vi "commander8.vi"() -> ()   [LabVIEW 2015]
uses:
  G_DATA.vi
  G_LCM.vi
  G_VEH.vi
  G_NAV.vi
  G_PATH.vi
  <vilib>/addons/control/pid/pid.llb/PID (DBL).vi
  G_SEN.vi
  <vilib>/addons/control/pid/NI_PID_pid.lvlib
panel:
  in  "handle":dbl
  in  "shifthold":dbl=0.02
  out "String":string="콜 서비스 대기 중"
  out "EURECAR_VISION":T1
  out "count":i32
  out "P2V Sign":picture[](array[picture])=[bytes[7530], bytes[7530], bytes[7530], bytes[7530]]
  out "Array 2":picture[](array[picture])
  out "sign 2":picture[](array[picture])
  out "sign":picture[](array[picture])
  in  "TTL":bool
  in  "Steering gain":dbl=0.8
  out "obs shift":dbl format="%.2f"
  in  "lane keep":bool
  in  "replay":bool
  in  "x":dbl min=-5.0 max=5.0 step=1.0
  out "display":u32=10
  out "control":u32=10
  out "update":bool=TRUE
  in  "save lcm":bool
  out "LCM Recv Data":string="GGA_2\t266\rSDT_GPS_DATA\t268\rGGA_1\t268\rRMC_2\t259\rRMC_1\t262\rEYE_RAW_T\t537\rPATH_T\t1344\rIBEO_2202_T\t672\rPOS_T\t3572\rCON_T\t4009\rCAN_T\t4707\r"
  out "GPS DATA 2":T2={"type"="WAAS", "x_lcc"=-395.2637182511565, "y_lcc"=-852.8277788987846, "latdev"=0.99, "londev"=0.99, "sats"=11, "gps_l1_ranges"=0, "gps_l1_mask_ranges"=0, "gps_l2_mask_ranges"=0, "Heading"=151.74409645131422, "lon"=127.35651, "lat"=36.36776, "time"="15:03:34.8", "hgps"=151.54, "lag"=0.0, "MAP"="KAIST"} {"lag" format="%#_5g"; "hgps" format="%#_5g"; "lat" format="%#_11g"; "lon" format="%#_11g"; "Heading" format="%#_5g"; "latdev" format="%#_4g"; "londev" format="%#_4g"}
  in  "Obs":bool=TRUE
  in  "Log":bool
  out "path":u32=10
  out "sensor":u32=10 format="%02.0f"
  out "Speed limit":dbl=20.0
  out "collision":bool
  in  "Load Path":bool
  in  "Max. Vel.":dbl=20.0 min=-5.0 max=120.0 step=5.0
  in  "RESET PATH":bool
  out "col":i16(graph)
  out "stop":bool
  in  "Reverse":bool
  in  "STOP":bool
  out "Waveform Chart 4":cluster{"auto":i16, "run":i16}(graph)={"auto"=1, "run"=0}
  out "Waveform Chart 3":cluster{"Steer_input":dbl, dbl, "handle":dbl}(graph)
  out "Waveform Chart 2":T3(graph)={"VS_des"=0.0, "VS_can"=31.498562500000002, "VS_des"=20.0}
  out "Heading":cluster{"Heading":dbl, "hgps":dbl}(graph)={"Heading"=151.74409645131422, "hgps"=151.54}
  out "XY Graph 2":cluster{"Y":dbl[], "Y":dbl[]}[](graph)=[{"Y"=[-395.3040396828474], "Y"=[-852.7527551292769]}, {"Y"=array[29298 elements], "Y"=array[29298 elements]}, {"Y"=array[29298 elements], "Y"=array[29298 elements]}, {"Y"=[-390.58210518912017], "Y"=[-861.284610912867]}]
  out "Gauge":cluster{dbl, dbl, dbl}(knob)={0.0, 31.498562500000002, 20.0} scale=-20.0..140.0
  out "Meter":cluster{dbl, dbl, dbl}(knob)={-3.5333877271700453, -5.2, -7.217874503679048} scale=-550.0..550.0
  out "XY Graph":cluster{"Y":dbl[], "Y":dbl[]}[](graph)=[{"Y"=array[11233 elements], "Y"=array[11233 elements]}, {"Y"=[-0.0, 0.0027755521495791413, 0.011103235155417224, 0.024986130588096955, 0.04442938073793812, 0.0694401981527264, 0.10002787904836907, 0.13620382065079895, 0.17798154254490584, 0.22537671212434418, 0.2784071742547809, 0.3370929852830926, 0.40145645154536425, 0.4715221725490224, 0.5473170890276435, 0.6288705360921867, 0.7162143017295008, 0.8093826909282242, 0.9084125957438758, 1.0133435716494645, 1.1242179205557647, 1.2410807809266515, 1.3639802254602955, 1.4929673668571652, 1.6280964722509026, 1.769425086939485, 1.9170141681219874, 2.0709282294217246, 2.2312354970611636, 2.3980080786478197, 2.5713221456362234], "Y"=[0.0, 0.5, 1.0, 1.5, 2.0, 2.5, 3.0, 3.5, 4.0, 4.5, 5.0, 5.5, 6.0, 6.5, 7.0, 7.5, 8.0, 8.5, 9.0, 9.5, 10.0, 10.5, 11.0, 11.5, 12.0, 12.5, 13.0, 13.5, 14.0, 14.5, 15.0]}, {"Y"=[-0.40885366553013214], "Y"=[0.1442103688222703]}, {"Y"=array[212 elements], "Y"=array[212 elements]}, {"Y"=[-0.925, -0.925, -0.925, -0.6775, -0.6775, -0.925, -0.925, -0.925, -0.925, -0.6775, -0.6775, -0.925, -0.925, -0.925, 0.9025, 0.9025, 0.9025, 0.6775, 0.6775, 0.9025, 0.9025, 0.9025, 0.9025, 0.6775, 0.6775, 0.9025, 0.9025, 0.9025, -0.925], "Y"=[-0.75, -0.224, 0.224, 0.224, -0.224, -0.224, 0.224, 2.415, 2.885, 2.885, 2.415, 2.415, 2.885, 3.5, 3.5, 2.885, 2.415, 2.415, 2.885, 2.885, 2.415, 0.224, -0.224, -0.224, 0.224, 0.224, -0.224, -0.75, -0.75]}, {"Y"=[0.0, 0.0, 0.0, 0.0, 0.0, 0.0, 0.0, 0.0, 0.0, 0.0], "Y"=[0.0, 0.5, 1.0, 1.5, 2.0, 2.5, 3.0, 3.5, 4.0, 4.5]}, {"Y"=[1.41796875, 1.3798326583616436, 1.3415997434556484, 1.3032752327956258, 1.2648643538951874, 1.226372334267944, 1.1878044014275073, 1.1491657828874886, 1.110461706161499, 1.07169739876315], "Y"=[0.0, 0.5, 1.0, 1.5, 2.0, 2.5, 3.0, 3.5, 4.0, 4.5]}, {"Y"=[-2.5234375, -2.5105986626297234, -2.4915998479127883, -2.466420726940036, -2.4350409708023073, -2.3974402505904435, -2.3535982373952864, -2.303494602307677, -2.247109016418457, -2.184421150818467], "Y"=[0.0, 0.5, 1.0, 1.5, 2.0, 2.5, 3.0, 3.5, 4.0, 4.5]}, {"Y"=[0.0, 0.0, 0.0, 0.0, 0.0, 0.0, 0.0, 0.0, 0.0, 0.0, 0.0, 0.0, 0.0, 0.0, 0.0, 0.0, 0.0, 0.0, 0.0, 0.0], "Y"=[0.0, 0.5, 1.0, 1.5, 2.0, 2.5, 3.0, 3.5, 4.0, 4.5, 5.0, 5.5, 6.0, 6.5, 7.0, 7.5, 8.0, 8.5, 9.0, 9.5]}]
  in  "Make WPT":bool
  # "e"
  # "V2I Traffic Signal"
  # "CNN\nSign\nDetection"
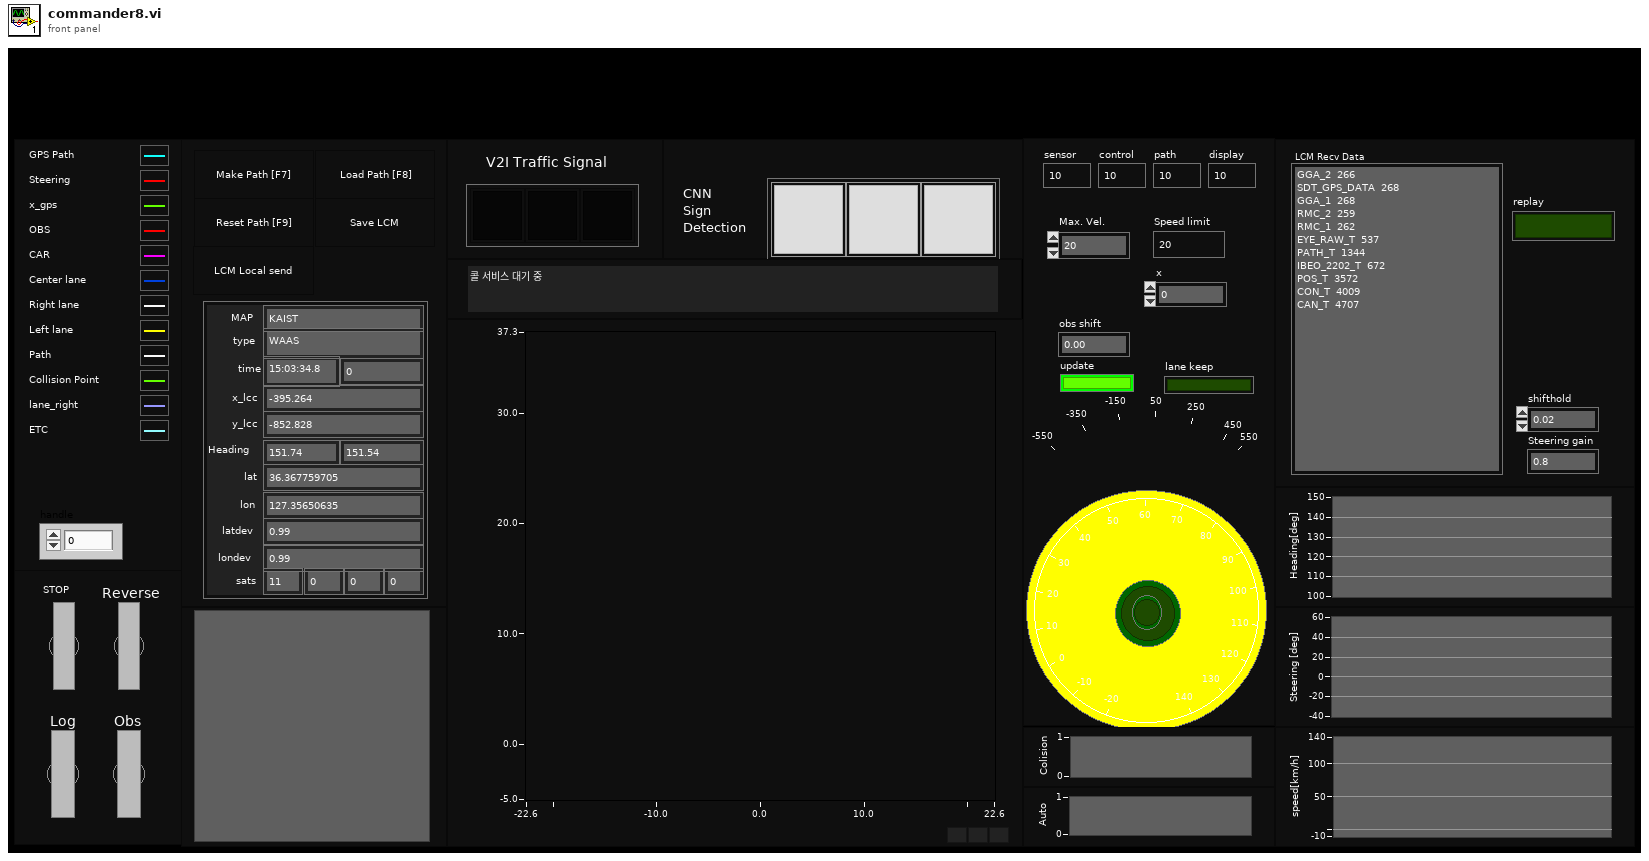
[diagram p1: front panel]
types:
  T1 = cluster{"hash":i64, "sys time":i64, "status":i32, "TS_num":i32, "TS_type":i32[], "TS_loc_x":dbl[], "TS_loc_y":dbl[]}
  T2 = cluster{"type":string, "x_lcc":dbl, "y_lcc":dbl, "latdev":sgl, "londev":sgl, "sats":u8, "gps_l1_ranges":u8, "gps_l1_mask_ranges":u8, "gps_l2_mask_ranges":u8, "Heading":dbl, "lon":sgl, "lat":sgl, "time":string, "hgps":dbl, "lag":dbl, "MAP":string}
  T3 = cluster{"VS_des":dbl, "VS_can":dbl, "VS_des":dbl}
  T4 = enum8{"Enabled", "Disabled", "Disabled and Grayed Out"}
  T5 = cluster{"proportional gain (Kc)":dbl, "integral time (Ti, min)":dbl, "derivative time (Td, min)":dbl}
  T6 = cluster{"idx":i32, "x":dbl, "y":dbl, "h":dbl, "x_path":dbl}
  T7 = cluster{"idx":i32, "x":dbl, "y":dbl, "hp":dbl, "x_path":dbl}
  T8 = cluster{"Steer_input":dbl, "Steer_output":dbl, "VS_des":dbl, "VS_can":dbl, "heading":dbl, "auto":bool, "run":bool, "x":dbl, "y":dbl}
  T9 = cluster{"GPSTime":dbl, "attitude[2]":dbl, "lcc[0]":dbl, "lcc[1]":dbl, "heading_GPS":dbl}
  T10 = cluster{"X":cluster{"idx":i32, "x":dbl, "y":dbl, "h":dbl, "x_path":dbl}}[]
  T11 = typedef "imagedata.ctl" = cluster{"image type":i32, "image depth":i32, "image":u8[], "mask":u8[], "colors":u32[], "Rectangle":cluster{"left":i16, "top":i16, "right":i16, "bottom":i16}}
  T12 = cluster{"hash":i64, "sys time":i64, "s_lat":dbl, "s_lon":dbl, "d_lat":dbl, "d_lon":dbl, "Message":i64}
  T13 = cluster{"Minimum":dbl, "Minimum":dbl, "Minimum":dbl, "Minimum":dbl, "Minimum":dbl}
  T14 = cluster{"X":cluster{"c_idx":i32, "xc":dbl, "yc":dbl, "hc":dbl, "xc_path":dbl}}[]
  T15 = cluster{"hash":i64, "sys time":i64, "time":dbl, "x":dbl, "y":dbl, "h":dbl, "numSV":i32, "postype":i32, "lag":i32, "hordev":dbl, "lat":dbl, "lon":dbl, "hgt":dbl, "map_idx":i32}
  T16 = cluster{"identifier":u32, "timestamp":timestamp, "payload":u8[]}
  T17 = cluster{"hash":i64, "sys time":i64, "size":i32, "data":u8[]}
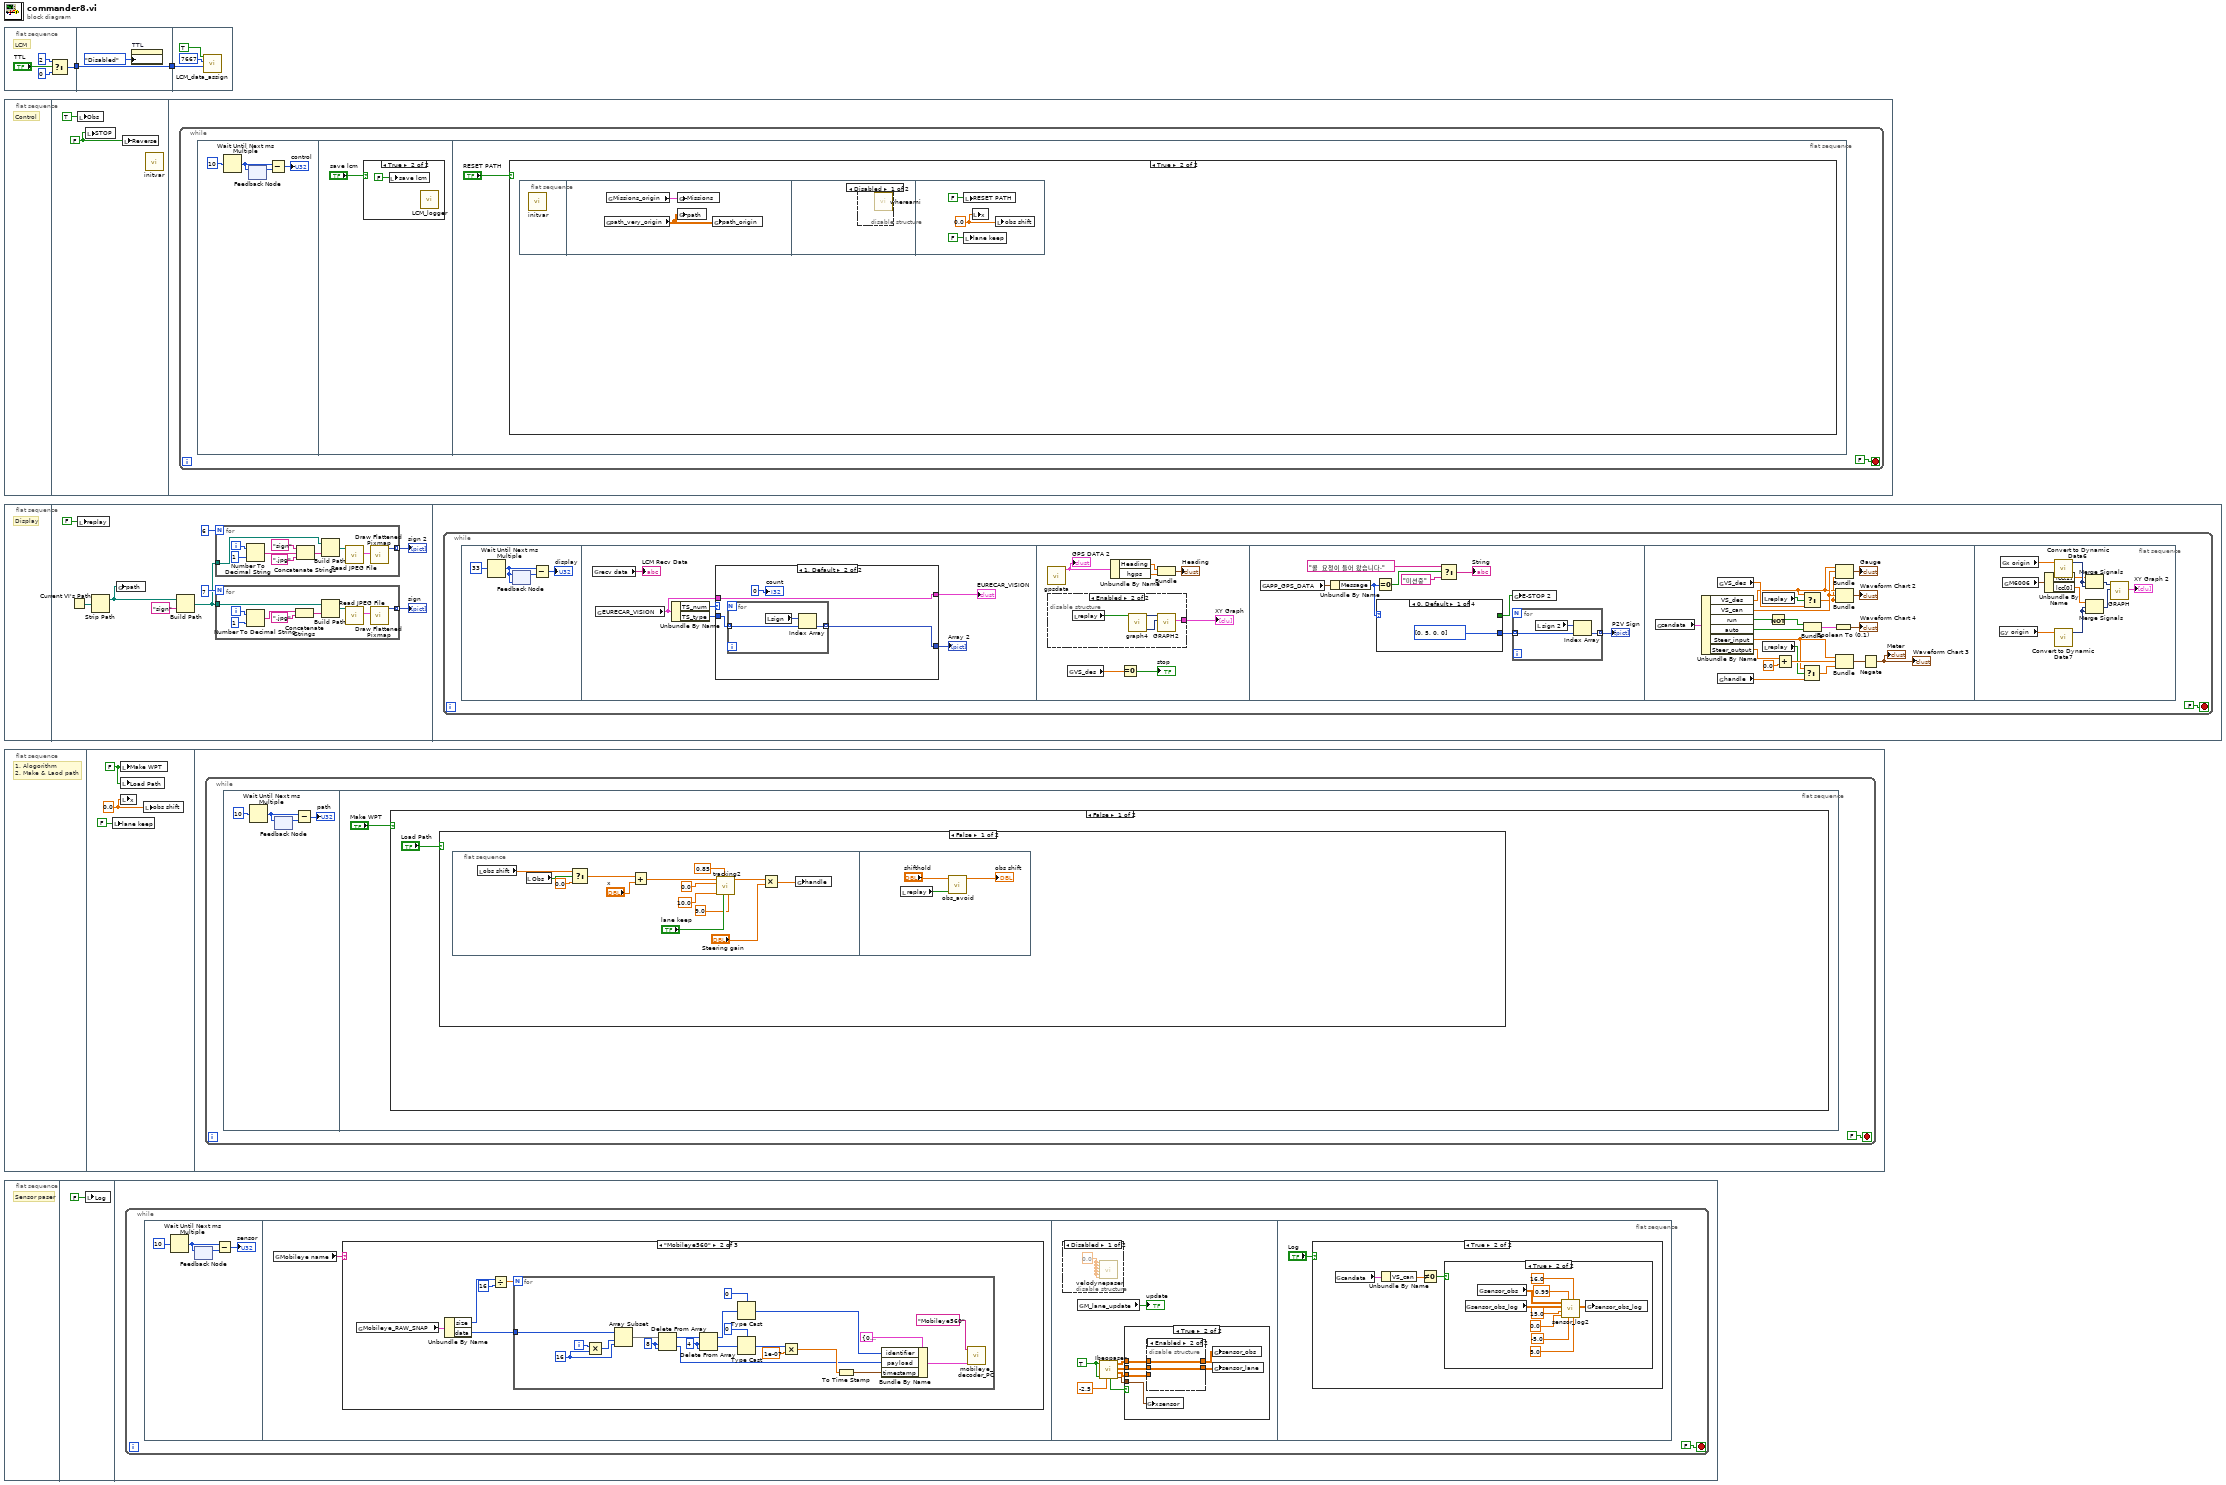
[diagram p0: block diagram]
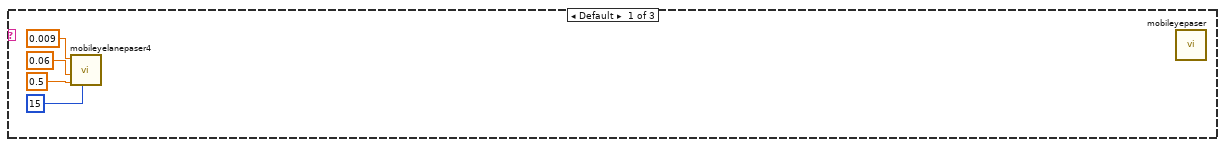
[diagram p2: hidden frame]
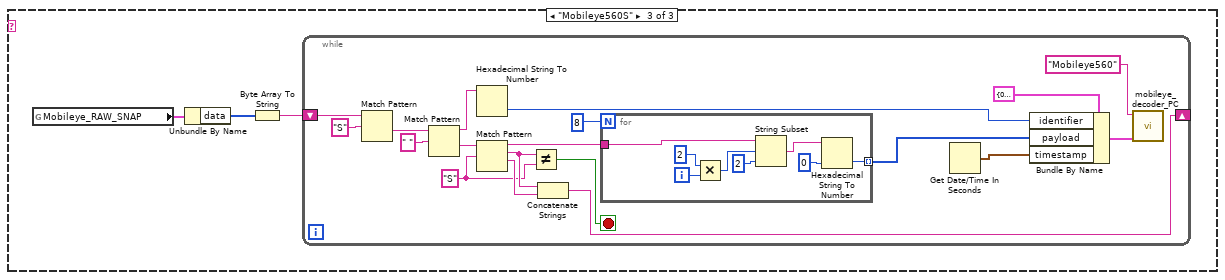
[diagram p3: hidden frame]
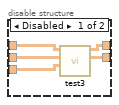
[diagram p6: hidden frame]
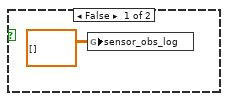
[diagram p7: hidden frame]
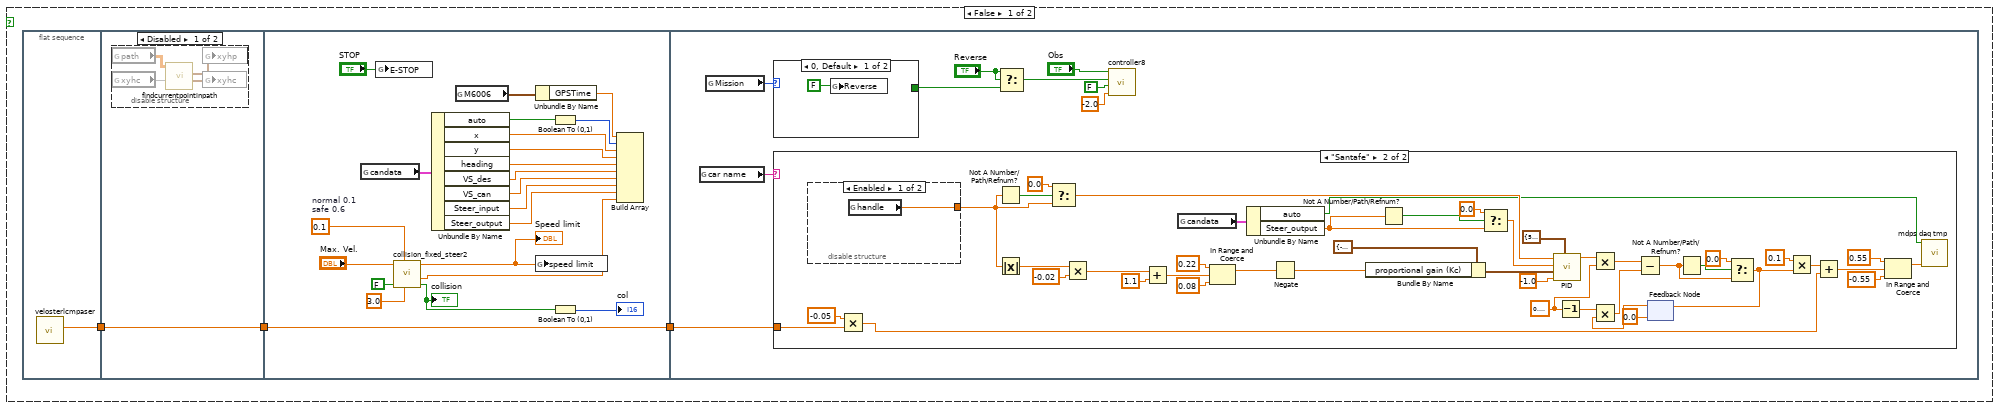
[diagram p10: hidden frame]
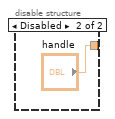
[diagram p13: hidden frame]
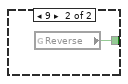
[diagram p14: hidden frame]
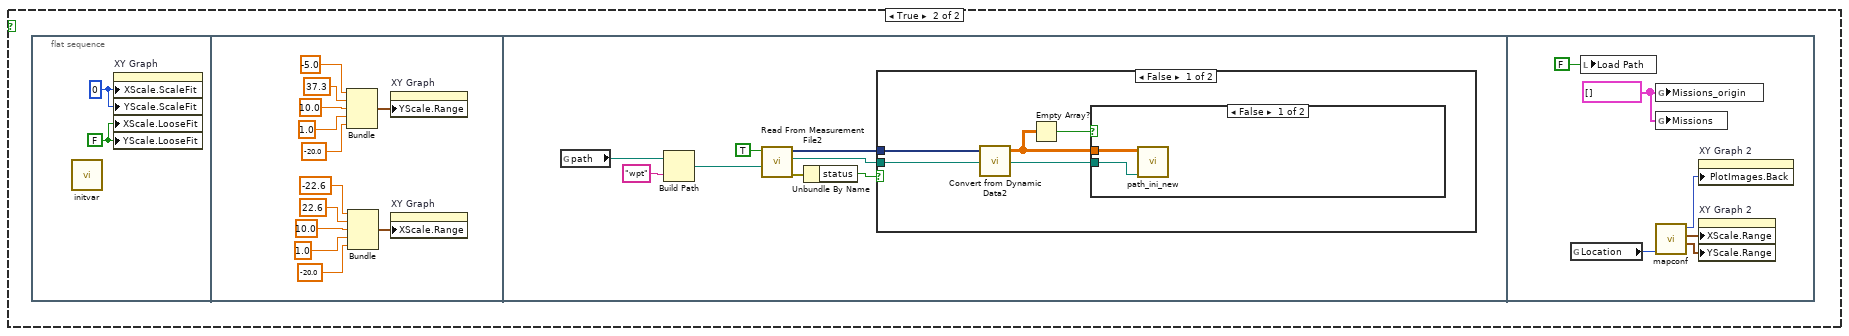
[diagram p16: hidden frame]
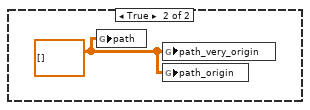
[diagram p17: hidden frame]
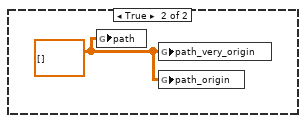
[diagram p18: hidden frame]
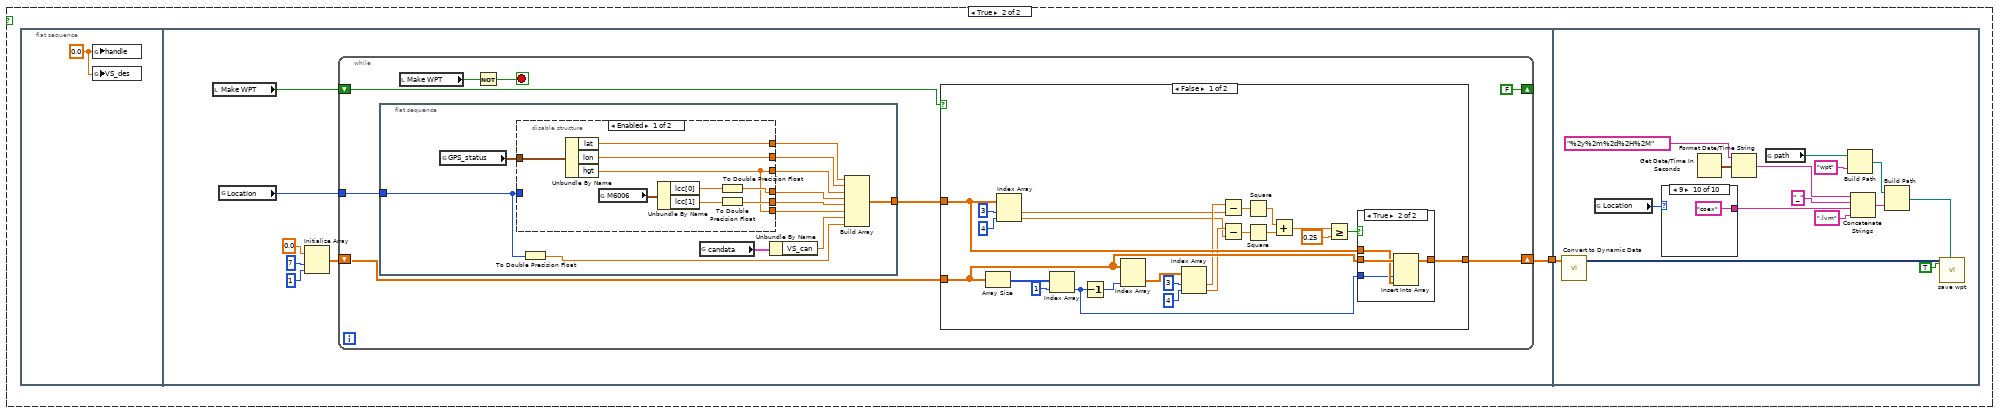
[diagram p19: hidden frame]
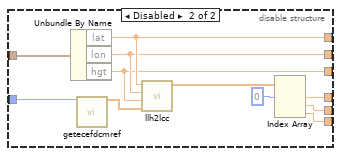
[diagram p20: hidden frame]
diagram:
  n1 = flat-sequence {
    tunnel: [w3] -> w1
    tunnel: [w8] -> w2
    tunnel: w1 -> [w8]
    tunnel: w2 -> [w11]
    frame #0 {
      # "LCM"
      n2 = Select(t=u16 2 ("time-to-live"), s="TTL", f=u16 0 ("time-to-live")) -> (s? t:f=w3:u16)
    }
    frame #1 {
      n3 = property on="TTL" class="Bool (strict)"("DisabledEnum"=T4."Disabled" ("Disabled")) -> ()  [unwired: 2 in, 2 out]
    }
    frame #2 {
      n4 = call "LCM_data_assign.vi"("time-to-live"=w11, "port"=u16 7667, "velodyne enable"=TRUE) -> ()  [unwired: 9 in]
    }
  }
  n5 = flat-sequence {
    frame #0 {
      # "Control"
    }
    frame #1 {
      w13 = FALSE ("LCM")
      n6 = local write "Obs"(TRUE ("obs")) -> ()
      n7 = local write "STOP"(w13) -> ()
      n8 = local write "Reverse"(w13) -> ()
      n9 = call "initvar.vi"() -> ()  [unwired: 12 in]
    }
    frame #2 {
      n10 = while {
        stop <- FALSE ("Loop 1") stop-if-true
        n11 = flat-sequence {
          frame #0 {
            n12 = Wait Until Next ms Multiple(millisecond multiple=u32 10 ("milliseconds to wait")) -> (millisecond timer value=w15:u32)
            n13 = feedback #1() -> (w16:u32)  [unwired: 1 in]
            n14 = feedback-in #1(w15) -> ()
            n15 = Subtract(x=w15, y=w16) -> (x-y=→"control":u32)
          }
          frame #1 {
            n16 = case shown="True" "save lcm" {
              frame False {
              }
              frame True {
                n17 = local write "save lcm"(FALSE ("save lcm")) -> ()
                n18 = call "LCM_logger.vi"() -> ()  [unwired: 12 in]
              }
            }
          }
          frame #2 {
            n19 = case shown="True" "RESET PATH" {
              frame False {
                n20 = flat-sequence {
                  tunnel: [w25] -> w24
                  tunnel: w24 -> [w26]
                  tunnel: [w26] -> w23
                  tunnel: w23 -> [w48]
                  tunnel: [w48] -> w22
                  tunnel: w22 -> [w55]
                  frame #0 {
                    n21 = call "velosterlcmpaser.vi"() -> ("mdps torque"=w25:dbl)  [unwired: 10 in, 1 out]
                  }
                  frame #1 {
                    n22 = disable-structure shown="Disabled" {
                      frame Disabled {
                        n23 = global read "G_PATH.vi" "path"() -> (w28:dbl[][])
                        n24 = global read "G_VEH.vi" "xyhc"() -> (w29)
                        n25 = call "findcurrentpointinpath.vi"("xyhc_in"=w29, "path_updated"=w28) -> ("xyhc_out"=w27:T6, "xyhp"=w30:T7)  [unwired: 8 in]
                        n26 = global write "G_VEH.vi" "xyhp"(w30) -> ()
                        n27 = global write "G_VEH.vi" "xyhc"(w27) -> ()
                      }
                      frame Enabled {
                      }
                    }
                  }
                  frame #2 {
                    w46 = 0.1  # normal 0.1 safe 0.6
                    n28 = global read "G_VEH.vi" "candata"() -> (w43:T8)
                    n29 = global write "G_VEH.vi" "E-STOP"("STOP") -> ()
                    n30 = call "collision_fixed_steer2.vi"("safe  dist"=3.0, "y"=w46, "obsclose"=FALSE, "Max. Vel."="Max. Vel.") -> ("collision"=w45:bool, "collision dist"=w31:dbl, "speed limit"=w44:dbl)  [unwired: 5 in]
                    "collision" <- w45
                    "Speed limit" <- w44
                    n31 = Unbundle By Name(w43) -> ("auto"=w33:bool, "x"=w42:dbl, "y"=w41:dbl, "heading"=w40:dbl, "VS_des"=w39:dbl, "VS_can"=w38:dbl, "Steer_input"=w37:dbl, "Steer_output"=w36:dbl)
                    n32 = global read "G_NAV.vi" "M6006"() -> (w35:T9)
                    n33 = Unbundle By Name(w35) -> ("GPSTime"=w34:dbl)
                    n34 = global write "G_VEH.vi" "speed limit"(w44) -> ()
                    n35 = Boolean To (0,1)(Boolean=w33) -> (0, 1=w32:i16)
                    n36 = Boolean To (0,1)(Boolean=w45) -> (0, 1=→"col":i16)
                    n37 = Build Array(w34, w32, w42, w41, w40, w39, w38, w37, w36, w31) -> ()  [unwired: 1 out]
                  }
                  frame #3 {
                    n38 = global read "G_LCM.vi" "car name"() -> (w56:string)
                    n39 = global read "G_PATH.vi" "Mission"() -> (w61:i32)
                    n40 = case shown="0, Default" w61 {
                      tunnel: [_ w108] -> w58
                      frame 0, Default {
                        n41 = global write "G_VEH.vi" "Reverse"(FALSE ("Reverse")) -> ()
                      }
                      frame 9 {
                        n42 = global read "G_VEH.vi" "Reverse"() -> (w108:bool)
                      }
                    }
                    n43 = case shown="\"Santafe\"" w56 {
                      tunnel: w55 -> [_ w95]
                      frame "False", Default {
                      }
                      frame "Santafe" {
                        w84 = 0.6000000000000001 ("y")
                        n44 = disable-structure shown="Enabled" {
                          disable-tunnel: [w105 "handle"] -> w62
                          frame Enabled {
                            n45 = global read "G_VEH.vi" "handle"() -> (w105:dbl)
                          }
                          frame Disabled {
                          }
                        }
                        n46 = Multiply(x=-0.05 ("x 5"), y=w95) -> (x*y=w93:dbl)
                        n47 = Not A Number/Path/Refnum?(number/path/refnum=w62) -> (NaN/Path/Refnum?=w87:bool)
                        n48 = Absolute Value(x=w62) -> (abs(x)=w78:dbl)
                        n49 = Select(t=0.0, s=w87, f=w62) -> (s? t:f=w86:dbl)
                        n50 = Multiply(x=w78, y=-0.02) -> (x*y=w76:dbl)
                        n51 = Add(x=w76, y=1.1) -> (x+y=w74:dbl)
                        n52 = global read "G_VEH.vi" "candata"() -> (w104:T8)
                        n53 = In Range and Coerce(upper limit=0.22, x=w74, lower limit=0.08) -> (coerced(x)=w71:dbl)  [unwired: 1 out]
                        n54 = Unbundle By Name(w104) -> ("auto"=w63:bool, "Steer_output"=w90:dbl)
                        n55 = Negate(x=w71) -> (-x=w69:dbl)
                        n56 = Bundle By Name(cluster=T5 {"proportional gain (Kc)"=-0.1, "integral time (Ti, min)"=0.0, "derivative time (Td, min)"=0.0} ("PID gains"), "proportional gain (Kc)"=w69) -> (w68:T5)
                        n57 = Not A Number/Path/Refnum?(number/path/refnum=w90) -> (NaN/Path/Refnum?=w92:bool)
                        n58 = Select(t=0.0, s=w92, f=w90) -> (s? t:f=w89:dbl)
                        n59 = call-poly <vilib>:"PID.vi"("output range"=cluster{"output high":dbl, "output low":dbl} {"output high"=5.0, "output low"=-5.0}, "dt (s)"=-1.0, "PID gains"=w68, "process variable"=w89, "setpoint"=w86) -> ("output"=w85:dbl)  [unwired: 5 in, 1 out]
                        n60 = Decrement(x=w84) -> (x-1=w83:dbl)
                        n61 = Multiply(x=w85, y=w84) -> (x*y=w80:dbl)
                        n62 = feedback #2(0.0) -> (w82:dbl)
                        n63 = Multiply(x=w83, y=w82) -> (x*y=w81:dbl)
                        n64 = Subtract(x=w80, y=w81) -> (x-y=w65:dbl)
                        n65 = Not A Number/Path/Refnum?(number/path/refnum=w65) -> (NaN/Path/Refnum?=w67:bool)
                        n66 = Select(t=0.0, s=w67, f=w65) -> (s? t:f=w64:dbl)
                        n67 = feedback-in #2(w64) -> ()
                        n68 = Multiply(x=0.1 ("x 2"), y=w64) -> (x*y=w94:dbl)
                        n69 = Add(x=w94, y=w93) -> (x+y=w101:dbl)
                        n70 = In Range and Coerce(upper limit=0.55, x=w101, lower limit=-0.55) -> (coerced(x)=w100:dbl)  [unwired: 1 out]
                        n71 = call "mdps daq tmp.vi"("steering"=w100, "auto"=w63) -> ()  [unwired: 10 in]
                      }
                    }
                    n72 = Select(t="Reverse", s="Reverse", f=w58) -> (s? t:f=w59:bool)
                    n73 = call "controller8.vi"("Neg max speed"=-2.0, "vel"=FALSE, "reverse"=w59, "obs"="Obs") -> ()  [unwired: 8 in]
                  }
                }
              }
              frame True {
                n74 = flat-sequence {
                  frame #0 {
                    n75 = call "initvar.vi"() -> ()  [unwired: 12 in]
                  }
                  frame #1 {
                    n76 = global read "G_PATH.vi" "path_very_origin"() -> (w110:dbl[][])
                    n77 = global read "G_PATH.vi" "Missions_origin"() -> (w109:T10)
                    n78 = global write "G_PATH.vi" "Missions"(w109) -> ()
                    n79 = global write "G_PATH.vi" "path"(w110) -> ()
                    n80 = global write "G_PATH.vi" "path_origin"(w110) -> ()
                  }
                  frame #2 {
                    n81 = disable-structure shown="Disabled" {
                      frame Disabled {
                        n82 = call "whereami.vi"() -> ()  [unwired: 12 in]
                      }
                      frame Enabled {
                      }
                    }
                  }
                  frame #3 {
                    w111 = 0.0 ("x")
                    n83 = local write "RESET PATH"(FALSE ("RESET PATH")) -> ()
                    n84 = local write "lane keep"(FALSE ("lane keep")) -> ()
                    n85 = local write "x"(w111) -> ()
                    n86 = local write "obs shift"(w111) -> ()
                  }
                }
              }
            }
          }
        }
      }
    }
  }
  n87 = flat-sequence {
    frame #0 {
      # "Display"
    }
    frame #1 {
      n88 = Current VI's Path() -> (path=w121:path)
      n89 = local write "replay"(FALSE ("replay")) -> ()
      n90 = Strip Path(path=w121) -> (stripped path=w114:path)  [unwired: 1 out]
      n91 = global write "G_DATA.vi" "path"(w114) -> ()
      n92 = Build Path(base path=w114, name or relative path="sign") -> (appended path=w115:path)
      n93 = for {
        N: 6 -> [_]
        tunnel: [w131] -> w117 mode=indexing
        tunnel: w115 -> [w126]
        i -> [w130]
        n94 = Number To Decimal String(number=w130, width (-)=i16 1) -> (decimal integer string=w128:string)
        n95 = Concatenate Strings("sign" ("string"), w128, ".jpg") -> (w125:string)
        n96 = Build Path(base path=w126, name or relative path=w125) -> (appended path=w124:path)
        n97 = call <vilib>:"Read JPEG File.vi"("path to JPEG file"=w124) -> ("image data"=w132:T11)  [unwired: 8 in, 2 out]
        n98 = call <vilib>:"Draw Flattened Pixmap.vi"("image data"=w132) -> ("new picture"=w131:picture)  [unwired: 8 in]
      }
      "sign 2" <- w117
      n99 = for {
        N: 7 -> [_]
        tunnel: [w140] -> w118 mode=indexing
        tunnel: w115 -> [w135]
        i -> [w139]
        n100 = Number To Decimal String(number=w139, width (-)=i16 1) -> (decimal integer string=w137:string)
        n101 = Concatenate Strings(w137, ".jpg") -> (w134:string)
        n102 = Build Path(base path=w135, name or relative path=w134) -> (appended path=w133:path)
        n103 = call <vilib>:"Read JPEG File.vi"("path to JPEG file"=w133) -> ("image data"=w141:T11)  [unwired: 8 in, 2 out]
        n104 = call <vilib>:"Draw Flattened Pixmap.vi"("image data"=w141) -> ("new picture"=w140:picture)  [unwired: 8 in]
      }
      "sign" <- w118
    }
    frame #2 {
      n105 = while {
        stop <- FALSE ("Loop 2") stop-if-true
        n106 = flat-sequence {
          frame #0 {
            n107 = Wait Until Next ms Multiple(millisecond multiple=u32 33 ("milliseconds to wait")) -> (millisecond timer value=w143:u32)
            n108 = feedback #3(w143) -> (w145:u32)
            n109 = feedback-in #3(w143) -> ()
            n110 = Subtract(x=w143, y=w145) -> (x-y=→"display":u32)
          }
          frame #1 {
            n111 = global read "G_LCM.vi" "recv data"() -> (→"LCM Recv Data":string)
            n112 = global read "G_LCM.vi" "EURECAR_VISION"() -> (w149:T1)
            n113 = Unbundle By Name(w149) -> ("TS_num"=w152:i32, "TS_type"=w151:i32[])
            n114 = case shown="1, Default" w152 {
              tunnel: w151 -> [_ w167]
              tunnel: [w160 w166] -> w150
              tunnel: w149 -> [_ w164]
              tunnel: [w153 w164] -> w148
              frame 0 {
                w162 = 100 ("x")
                n115 = local read "count"() -> (w163:i32)
                n116 = Increment(x=w163) -> (x+1=w158:i32)
                n117 = Max & Min(x=w162, y=w158) -> (min(x,y)=w157:i32)  [unwired: 1 out]
                n118 = local read "EURECAR_VISION"() -> (w154:T1)
                n119 = local write "count"(w157) -> ()
                n120 = Equal?(x=w162, y=w157) -> (x = y?=w156:bool)
                n121 = local read "Array 2"() -> (w159:picture[])
                n122 = Select(t=T1 {"hash"=0, "sys time"=0, "status"=0, "TS_num"=0, "TS_type"=[], "TS_loc_x"=[], "TS_loc_y"=[]} ("EURECAR_VISION"), s=w156, f=w154) -> (s? t:f=w153:T1)
                n123 = Select(t=picture[] [], s=w156, f=w159) -> (s? t:f=w160:picture[])
              }
              frame 1, Default {
                n124 = for {
                  tunnel: w167 -> [w169] mode=indexing
                  tunnel: [w168] -> w166 mode=indexing
                  n125 = local read "sign"() -> (w170:picture[])
                  n126 = Index Array(array=w170, index=w169) -> (element=w168:picture)
                }
                "count" <- 0 ("Numeric Control")
              }
            }
            "Array 2" <- w150
            "EURECAR_VISION" <- w148
          }
          frame #2 {
            n127 = call "gpsdata.vi"() -> ("GPS DATA 2"=w173:T2)  [unwired: 11 in]
            "GPS DATA 2" <- w173
            n128 = disable-structure shown="Enabled" {
              disable-tunnel: [w178 w183] -> w171
              frame Disabled {
                n129 = call "graph3.vi"("replay"="replay") -> ("XY Graph"=w178:cluster{"Y":dbl[], "Y":dbl[]}[])  [unwired: 9 in, 1 out]
              }
              frame Enabled {
                n130 = local read "replay"() -> (w180:bool)
                n131 = call "graph4.vi"("replay"=w180) -> ("y"=w181:dynamicdata, "x"=w182:dynamicdata)  [unwired: 9 in]
                n132 = call "GRAPH2"("Y Input"=w181, "X Input"=w182) -> ("XY Graph"=w183:cluster{"Y":dbl[], "Y":dbl[]}[])  [unwired: 3 in, 6 out]
              }
            }
            "XY Graph" <- w171
            n133 = global read "G_VEH.vi" "VS_des"() -> (w177:dbl)
            n134 = Unbundle By Name(w173) -> ("Heading"=w175:dbl, "hgps"=w174:dbl)
            n135 = Equal To 0?(x=w177) -> (x = 0?=→"stop":bool)
            n136 = Bundle("Heading"=w175, "hgps"=w174) -> (→"Heading":cluster{"Heading":dbl, "hgps":dbl})  [unwired: 1 in]
          }
          frame #3 {
            n137 = global read "G_LCM.vi" "APP_GPS_DATA"() -> (w189:T12)
            n138 = Unbundle By Name(w189) -> ("Message"=w188:i64)
            n139 = Equal To 0?(x=w188) -> (x = 0?=w187:bool)
            n140 = case shown="0, Default" w188 {
              tunnel: [_ TRUE _ _] -> w192
              tunnel: [i32[] [0, 5, 0, 0] i32[] [1, 5, 0, 0] i32[] [0, 2, 0, 0] i32[] [0, 5, 3, 0]] -> w191
              frame 0, Default {
              }
              frame 1 {
              }
              frame 2 {
              }
              frame 3 {
              }
            }
            n141 = Select(t="콜  요청이 들어 왔습니다.", s=w187, f="미션중") -> (s? t:f=→"String":string)
            n142 = global write "G_VEH.vi" "E-STOP 2"(w192) -> ()
            n143 = for {
              tunnel: w191 -> [w199] mode=indexing
              tunnel: [w198] -> w190 mode=indexing
              n144 = local read "sign 2"() -> (w200:picture[])
              n145 = Index Array(array=w200, index=w199) -> (element=w198:picture)
            }
            "P2V Sign" <- w190
          }
          frame #4 {
            n146 = global read "G_VEH.vi" "candata"() -> (w222:T8)
            n147 = Unbundle By Name(w222) -> ("VS_des"=w203:dbl, "VS_can"=w215:dbl, "run"=w213:bool, "auto"=w214:bool, "Steer_input"=w207:dbl, "Steer_output"=w212:dbl)
            n148 = global read "G_VEH.vi" "VS_des"() -> (w204:dbl)
            n149 = global read "G_VEH.vi" "handle"() -> (w208:dbl)
            n150 = local read "replay"() -> (w205:bool)
            n151 = local read "replay"() -> (w209:bool)
            n152 = Not(x=w213) -> (.not. x?=w217:bool)
            n153 = Add(x=w212, y=0.0) -> (x+y=w210:dbl)
            n154 = Select(t=w207, s=w209, f=w208) -> (s? t:f=w206:dbl)
            n155 = Select(t=w203, s=w205, f=w204) -> (s? t:f=w202:dbl)
            n156 = Bundle(w217, "auto"=w214) -> (w219:cluster{bool, "auto":bool})  [unwired: 1 in]
            n157 = Boolean To (0,1)(Boolean=w219) -> (0, 1=→"Waveform Chart 4":cluster{i16, "auto":i16})
            n158 = Bundle("VS_des"=w203, "VS_can"=w215, "VS_des"=w202) -> (→"Gauge":T3)  [unwired: 1 in]
            n159 = Bundle("VS_des"=w203, "VS_can"=w215, "VS_des"=w202) -> (→"Waveform Chart 2":T3)  [unwired: 1 in]
            n160 = Bundle("Steer_input"=w207, w210, "handle"=w206) -> (w221:cluster{"Steer_input":dbl, dbl, "handle":dbl})  [unwired: 1 in]
            n161 = Negate(x=w221) -> (-x=→"Meter" →"Waveform Chart 3":cluster{"Steer_input":dbl, dbl, "handle":dbl})
          }
          frame #5 {
            n162 = global read "G_PATH.vi" "y origin"() -> (w225:dbl[])
            n163 = global read "G_PATH.vi" "x origin"() -> (w226:dbl[])
            n164 = global read "G_NAV.vi" "M6006"() -> (w228:T9)
            n165 = Unbundle By Name(w228) -> ("lcc[1]"=w229:dbl, "lcc[0]"=w230:dbl)
            n166 = call "Convert to Dynamic Data6"("Array"=w226) -> ("Dynamic Data Type"=w232:dynamicdata)  [unwired: 3 in]
            n167 = call "Convert to Dynamic Data7"("Array"=w225) -> ("Dynamic Data Type"=w231:dynamicdata)  [unwired: 3 in]
            n168 = Merge Signals(w229, w232, w232) -> (w224:dynamicdata)
            n169 = Merge Signals(w230, w231, w231) -> (w223:dynamicdata)
            n170 = call "GRAPH"("Y Input"=w223, "X Input"=w224) -> ("XY Graph"=→"XY Graph 2":cluster{"Y":dbl[], "Y":dbl[]}[])  [unwired: 3 in, 6 out]
          }
        }
      }
    }
  }
  n171 = flat-sequence {
    frame #0 {
      # "1. Alogorithm\n2. Make & Laod path"
    }
    frame #1 {
      w233 = 0.0 ("x")
      w235 = FALSE ("Make WPT")
      n172 = local write "lane keep"(FALSE ("lane update")) -> ()
      n173 = local write "Make WPT"(w235) -> ()
      n174 = local write "Load Path"(w235) -> ()
      n175 = local write "x"(w233) -> ()
      n176 = local write "obs shift"(w233) -> ()
    }
    frame #2 {
      n177 = while {
        stop <- FALSE ("Loop 3") stop-if-true
        n178 = flat-sequence {
          frame #0 {
            n179 = Wait Until Next ms Multiple(millisecond multiple=u32 10 ("milliseconds to wait")) -> (millisecond timer value=w237:u32)
            n180 = feedback #4() -> (w239:u32)  [unwired: 1 in]
            n181 = feedback-in #4(w237) -> ()
            n182 = Subtract(x=w237, y=w239) -> (x-y=→"path":u32)
          }
          frame #1 {
            n183 = case shown="False" "Make WPT" {
              frame False {
                n184 = case shown="False" "Load Path" {
                  frame False {
                    n185 = flat-sequence {
                      frame #0 {
                        n186 = local read "obs shift"() -> (w245:dbl)
                        n187 = local read "Obs"() -> (w246:bool)
                        n188 = Select(t=w245, s=w246, f=0.0) -> (s? t:f=w243:dbl)
                        n189 = Add(x=w243, y="x") -> (x+y=w256:dbl)
                        n190 = call "tracking2.vi"("x 2"=9.0, "lane keep"="lane keep", "str_gain"=0.85, "Numeric 2"=10.0, "xbody"=0.0, "xt"=w256) -> ("handle"=w253:dbl)  [unwired: 4 in, 1 out]
                        n191 = Multiply(x=w253, y="Steering gain") -> (x*y=w255:dbl)
                        n192 = global write "G_VEH.vi" "handle"(w255) -> ()
                      }
                      frame #1 {
                        n193 = local read "replay"() -> (w257:bool)
                        n194 = call "obs_avoid.vi"("replay"=w257, "shifthold"="shifthold") -> ("obs shift"=→"obs shift":dbl)  [unwired: 9 in]
                      }
                    }
                  }
                  frame True {
                    n195 = flat-sequence {
                      frame #0 {
                        w261 = FALSE ("X Scale.Loose Fit")
                        w260 = u8 0 ("X Scale.Scale Fit")
                        n196 = call "initvar.vi"() -> ()  [unwired: 12 in]
                        n197 = property on="XY Graph" class="XYGraph (strict)"("XScale.ScaleFit"=w260, "YScale.ScaleFit"=w260, "XScale.LooseFit"=w261, "YScale.LooseFit"=w261) -> ()  [unwired: 2 in, 2 out]
                      }
                      frame #1 {
                        n198 = Bundle("Minimum"=-5.0, "Minimum"=37.3, "Minimum"=10.0, "Minimum"=1.0, "Minimum"=-20.0) -> (w266:T13)  [unwired: 1 in]
                        n199 = Bundle("Minimum"=-22.6, "Minimum"=22.6, "Minimum"=10.0, "Minimum"=1.0, "Minimum"=-20.0) -> (w273:T13)  [unwired: 1 in]
                        n200 = property on="XY Graph" class="XYGraph (strict)"("YScale.Range"=w266) -> ()  [unwired: 2 in, 2 out]
                        n201 = property on="XY Graph" class="XYGraph (strict)"("XScale.Range"=w273) -> ()  [unwired: 2 in, 2 out]
                      }
                      frame #2 {
                        n202 = global read "G_DATA.vi" "path"() -> (w277:path)
                        n203 = Build Path(base path=w277, name or relative path="wpt") -> (appended path=w275:path)
                        n204 = call "Read From Measurement File2"("Filename"=w275, "Reset"=TRUE) -> ("error out"=w279:errorcluster, "Filename Out"=w274:path, "Signals"=w281:dynamicdata)  [unwired: 4 in, 3 out]
                        n205 = Unbundle By Name(w279) -> ("status"=w278:bool)
                        n206 = case shown="False" w278 {
                          tunnel: w281 -> [w283 _]
                          tunnel: w274 -> [w282 _]
                          frame False {
                            n207 = call "Convert from Dynamic Data2"("Dynamic Data Type"=w283) -> ("Array"=w285:dbl[][])  [unwired: 3 in]
                            n208 = Empty Array?(array=w285) -> (empty?=w284:bool)
                            n209 = case shown="False" w284 {
                              tunnel: w285 -> [w287 _]
                              tunnel: w282 -> [w286 _]
                              frame False {
                                n210 = call "path_ini_new.vi"("Filename Out"=w286, "WPT"=w287) -> ()  [unwired: 10 in]
                              }
                              frame True {
                                w288 = dbl[][] [] ("path_updated")
                                n211 = global write "G_PATH.vi" "path"(w288) -> ()
                                n212 = global write "G_PATH.vi" "path_very_origin"(w288) -> ()
                                n213 = global write "G_PATH.vi" "path_origin"(w288) -> ()
                              }
                            }
                          }
                          frame True {
                            w289 = dbl[][] [] ("path_updated")
                            n214 = global write "G_PATH.vi" "path"(w289) -> ()
                            n215 = global write "G_PATH.vi" "path_very_origin"(w289) -> ()
                            n216 = global write "G_PATH.vi" "path_origin"(w289) -> ()
                          }
                        }
                      }
                      frame #3 {
                        w290 = T14 [] ("Missions_origin")
                        n217 = global read "G_VEH.vi" "Location"() -> (w291:i32)
                        n218 = local write "Load Path"(FALSE ("Load WPT")) -> ()
                        n219 = global write "G_PATH.vi" "Missions_origin"(w290) -> ()
                        n220 = global write "G_PATH.vi" "Missions"(w290) -> ()
                        n221 = call "mapconf.vi"("Location"=w291) -> ("y"=w293:cluster{dbl, dbl, "y":dbl, "y":dbl, dbl}, "x"=w294:cluster{dbl, dbl, "y":dbl, "y":dbl, dbl}, "new picture"=w295:picture)  [unwired: 8 in]
                        n222 = property on="XY Graph 2" class="XYGraph (strict)"("PlotImages.Back"=w295) -> ()  [unwired: 2 in, 2 out]
                        n223 = property on="XY Graph 2" class="XYGraph (strict)"("XScale.Range"=w294, "YScale.Range"=w293) -> ()  [unwired: 2 in, 2 out]
                      }
                    }
                  }
                }
              }
              frame True {
                n224 = flat-sequence {
                  tunnel: [w300] -> w296
                  tunnel: w296 -> [w389]
                  frame #0 {
                    w297 = 0.0
                    n225 = global write "G_VEH.vi" "handle"(w297) -> ()
                    n226 = global write "G_VEH.vi" "VS_des"(w297) -> ()
                  }
                  frame #1 {
                    n227 = local read "Make WPT"() -> (w299:bool)
                    n228 = global read "G_VEH.vi" "Location"() -> (w298:i32)
                    n229 = Initialize Array(0.0 ("element"), 7 ("dimension size"), 1 ("dimension size")) -> (w301:dbl[][])
                    n230 = while {
                      shift-right: [w306] -> w300
                      shift-left: w301 -> [w308]
                      shift-right: [FALSE] -> _
                      shift-left: w299 -> [w309]
                      tunnel: w298 -> [w305]
                      stop <- w311 stop-if-true
                      n231 = flat-sequence {
                        tunnel: [w321] -> w307
                        tunnel: w305 -> [w314]
                        frame #0 {
                          n232 = global read "G_NAV.vi" "GPS_status"() -> (w313:T15)
                          n233 = disable-structure shown="Enabled" {
                            disable-tunnel: [w332 w336] -> w324
                            disable-tunnel: [w331 w335] -> w323
                            disable-tunnel: [w325 w334] -> w322
                            disable-tunnel: w313 -> [w330 w344]
                            disable-tunnel: [w329 w343] -> w320
                            disable-tunnel: [w328 w342] -> w319
                            disable-tunnel: [w325 w341] -> w318
                            disable-tunnel: w314 -> [_ w340]
                            frame Enabled {
                              n234 = Unbundle By Name(w330) -> ("lat"=w329:dbl, "lon"=w328:dbl, "hgt"=w325:dbl)
                              n235 = global read "G_NAV.vi" "M6006"() -> (w333:T9)
                              n236 = Unbundle By Name(w333) -> ("lcc[0]"=w327:dbl, "lcc[1]"=w326:dbl)
                              n237 = To Double Precision Float(number=w327) -> (double precision float=w332:dbl)
                              n238 = To Double Precision Float(number=w326) -> (double precision float=w331:dbl)
                            }
                            frame Disabled {
                              n239 = Unbundle By Name(w344) -> ("lat"=w343:dbl, "lon"=w342:dbl, "hgt"=w341:dbl)
                              n240 = call "getecefdcmref.vi"("map name"=w340) -> ("XYZ"=w339:dbl[])  [unwired: 10 in, 4 out]
                              n241 = call "llh2lcc.vi"("ecef ref"=w339, "hgt"=w341, "lon"=w342, "lat"=w343) -> ("lcc"=w338:dbl[])  [unwired: 7 in]
                              n242 = Index Array(array=w338, index #1=0 ("index")) -> (element #1=w336:dbl, element #2=w335:dbl, element #3=w334:dbl)  [unwired: 2 in]
                            }
                          }
                          n243 = To Double Precision Float(number=w314) -> (double precision float=w315:dbl)
                          n244 = global read "G_VEH.vi" "candata"() -> (w317:T8)
                          n245 = Unbundle By Name(w317) -> ("VS_can"=w316:dbl)
                          n246 = Build Array(w320, w319, w318, w324, w323, w322, w316, w315) -> (w321:dbl[])
                        }
                      }
                      n247 = local read "Make WPT"() -> (w312:bool)
                      n248 = Not(x=w312) -> (.not. x?=w311:bool)
                      n249 = case shown="False" w309 {
                        tunnel: w308 -> [w359 w376]
                        tunnel: w307 -> [w358 w374]
                        tunnel: [w357 w373] -> w306
                        frame False {
                          n250 = Array Size(array=w359) -> (size(s)=w367:i32[])
                          n251 = Index Array(array=w358, index #1=3 ("index"), index #2=4 ("index")) -> (element #1=w353:dbl, element #2=w351:dbl)
                          n252 = Index Array(array=w367, index=1) -> (element=w356:i32)
                          n253 = Decrement(x=w356) -> (x-1=w355:i32)
                          n254 = Index Array(array=w359, index (col)=w355) -> (element=w363:dbl[])  [unwired: 1 in]
                          n255 = Index Array(array=w363, index #1=3 ("index"), index #2=4 ("index")) -> (element #1=w354:dbl, element #2=w352:dbl)
                          n256 = Subtract(x=w354, y=w353) -> (x-y=w350:dbl)
                          n257 = Subtract(x=w352, y=w351) -> (x-y=w349:dbl)
                          n258 = Square(x=w350) -> (x^2=w348:dbl)
                          n259 = Square(x=w349) -> (x^2=w347:dbl)
                          n260 = Add(x=w348, y=w347) -> (x+y=w346:dbl)
                          n261 = Greater Or Equal?(x=w346, y=0.25) -> (x >= y?=w360:bool)
                          n262 = case shown="True" w360 {
                            tunnel: w359 -> [w368 w372]
                            tunnel: w356 -> [_ w369]
                            tunnel: w358 -> [_ w371]
                            tunnel: [w368 w370] -> w357
                            frame False {
                            }
                            frame True {
                              n263 = Insert Into Array(array=w372, index (col)=w369, new element=w371) -> (w370:dbl[][])  [unwired: 1 in]
                            }
                          }
                        }
                        frame True {
                          n264 = Replace Array Subset(array=w376, new element=w374, index (col)=0 ("disabled index (col)")) -> (w373:dbl[][])  [unwired: 1 in]
                        }
                      }
                    }
                  }
                  frame #2 {
                    n265 = call "Convert to Dynamic Data"("2D Array"=w389) -> ("Dynamic Data Type"=w390:dynamicdata)  [unwired: 3 in]
                    n266 = global read "G_VEH.vi" "Location"() -> (w386:i32)
                    n267 = case shown="9" w386 {
                      tunnel: ["" ("String") "Hyundai" ("String") "KAIST" ("String") "AJOU" ("String") "MUNJI" ("String") "Airforce" ("String") "CAR" ("String") "KATRI" ("String") _ "coex" ("String")] -> w385
                      frame 0, Default {
                      }
                      frame 1 {
                      }
                      frame 2 {
                      }
                      frame 3 {
                      }
                      frame 4 {
                      }
                      frame 5 {
                      }
                      frame 6 {
                      }
                      frame 7 {
                      }
                      frame 8 {
                      }
                      frame 9 {
                      }
                    }
                    n268 = Get Date/Time In Seconds() -> (seconds since 1Jan1904=w387:timestamp)
                    n269 = Format Date/Time String(time format string (%c)="%2y%2m%2d%2H%2M", seconds (now)=w387) -> (date/time string=w383:string)  [unwired: 1 in]
                    n270 = global read "G_DATA.vi" "path"() -> (w381:path)
                    n271 = Build Path(base path=w381, name or relative path="wpt") -> (appended path=w379:path)
                    n272 = Concatenate Strings(w383, "_" ("string"), w385, ".lvm" ("string")) -> (w378:string)
                    n273 = Build Path(base path=w379, name or relative path=w378) -> (appended path=w377:path)
                    n274 = call "save wpt"("Signals"=w390, "Reset"=TRUE, "Filename"=w377) -> ()  [unwired: 14 in, 3 out]
                  }
                }
              }
            }
          }
        }
      }
    }
  }
  n275 = flat-sequence {
    frame #0 {
      # "Sensor paser"
    }
    frame #1 {
      n276 = local write "Log"(FALSE ("obs")) -> ()
    }
    frame #2 {
      n277 = while {
        stop <- FALSE ("Loop 4") stop-if-true
        n278 = flat-sequence {
          frame #0 {
            n279 = Wait Until Next ms Multiple(millisecond multiple=u32 10 ("milliseconds to wait")) -> (millisecond timer value=w403:u32)
            n280 = feedback #5() -> (w405:u32)  [unwired: 1 in]
            n281 = feedback-in #5(w403) -> ()
            n282 = Subtract(x=w403, y=w405) -> (x-y=→"sensor":u32)
          }
          frame #1 {
            n283 = global read "G_LCM.vi" "Mobileye name"() -> (w407:string)
            n284 = case shown="\"Mobileye560\"" w407 {
              frame Default {
                n285 = call "mobileyelanepaser4.vi"("count hold"=u64 15, "thresh  c"=0.5, "thresh  b"=0.06 ("thresh 2"), "thresh r"=0.009 ("y")) -> ()  [unwired: 4 in, 4 out]
                n286 = call "mobileyepaser.vi"() -> ()  [unwired: 11 in, 1 out]
              }
              frame "Mobileye560" {
                n287 = global read "G_LCM.vi" "Mobileye_RAW_SNAP"() -> (w412:T17)
                n288 = Unbundle By Name(w412) -> ("size"=w413:i32, "data"=w416:u8[])
                n289 = Divide(x=w413, y=16) -> (x/y=w415:dbl)
                n290 = for {
                  N: w415 -> [_]
                  tunnel: w416 -> [w437]
                  i -> [w436]
                  w429 = 4 ("length")
                  w427 = 8 ("index")
                  w435 = 16 ("y")
                  n291 = Multiply(x=w436, y=w435) -> (x*y=w434:i32)
                  n292 = Array Subset(array=w437, index=w434, length=w435) -> (w419:u8[])
                  n293 = Delete From Array(array=w419, length=w427, index=w427) -> (deleted portion=w420:u8[], array with subset deleted=w428:u8[])
                  n294 = Delete From Array(array=w428, length=w429, index=w429) -> (deleted portion=w433:u8[], array with subset deleted=w430:u8[])
                  n295 = Type Cast(type=u32 0, x=w430) -> (*(type *) &x=w421:u32)
                  n296 = Type Cast(type=u32 0, x=w433) -> (*(type *) &x=w422:u32)
                  n297 = Multiply(x=w422, y=1e-07) -> (x*y=w425:dbl)
                  n298 = To Time Stamp(1:w425) -> (0:w424:timestamp)
                  n299 = Bundle By Name(cluster=T16 {"identifier"=0, "timestamp"=timestamp(0 s since 1904-01-01), "payload"=[]} ("can cluster"), "identifier"=w421, "payload"=w420, "timestamp"=w424) -> (w418:T16)
                  n300 = call "mobileye_decoder_PC.vi"("can cluster"=w418, "name"="Mobileye560") -> ()  [unwired: 10 in]
                }
              }
              frame "Mobileye560S" {
                n301 = global read "G_LCM.vi" "Mobileye_RAW_SNAP"() -> (w440:T17)
                n302 = Unbundle By Name(w440) -> ("data"=w439:u8[])
                n303 = Byte Array To String(unsigned byte array=w439) -> (string=w438:string)
                n304 = while {
                  shift-right: [w443] -> _
                  shift-left: w438 -> [w445]
                  stop <- w444 stop-if-true
                  w449 = "S" ("regular expression")
                  n305 = Match Pattern(string=w445, regular expression="S") -> (after substring=w458:string)  [unwired: 1 in, 3 out]
                  n306 = Match Pattern(string=w458, regular expression=" ") -> (before substring=w456:string, after substring=w454:string)  [unwired: 1 in, 2 out]
                  n307 = Hexadecimal String To Number(string=w456) -> (number=w447:u32)  [unwired: 2 in, 1 out]
                  n308 = Match Pattern(string=w454, regular expression=w449) -> (before substring=w453:string, match substring=w450:string, after substring=w451:string)  [unwired: 1 in, 1 out]
                  n309 = Not Equal?(x=w450, y=w449) -> (x != y?=w444:bool)
                  n310 = Concatenate Strings(w450, w451) -> (w443:string)
                  n311 = for {
                    N: 8 -> [_]
                    tunnel: w453 -> [w467]
                    tunnel: [w463] -> w446 mode=indexing
                    i -> [w462]
                    n312 = Multiply(x=2, y=w462) -> (x*y=w465:i32)
                    n313 = String Subset(string=w467, offset (0)=w465, length (rest)=2 ("length (rest)")) -> (substring=w460:string)
                    n314 = Hexadecimal String To Number(string=w460, default (0uL)=u8 0) -> (number=w463:u8)  [unwired: 1 in, 1 out]
                  }
                  n315 = Get Date/Time In Seconds() -> (seconds since 1Jan1904=w452:timestamp)
                  n316 = Bundle By Name(cluster=T16 {"identifier"=0, "timestamp"=timestamp(0 s since 1904-01-01), "payload"=[]} ("can cluster"), "identifier"=w447, "payload"=w446, "timestamp"=w452) -> (w441:T16)
                  n317 = call "mobileye_decoder_PC.vi"("can cluster"=w441, "name"="Mobileye560") -> ()  [unwired: 10 in]
                }
              }
            }
          }
          frame #2 {
            w470 = TRUE ("Sensor [F12]")
            n318 = disable-structure shown="Disabled" {
              frame Disabled {
                w476 = 0.0 ("roll")
                n319 = call "velodynepaser.vi"("roll"=w476, "pitch"=w476, "heading"=w476, "dX"=w476, "dY"=w476, "dZ"=w476) -> ()  [unwired: 12 in, 2 out]
              }
              frame Enabled {
              }
            }
            n320 = global read "G_SEN.vi" "M_lane_update"() -> (→"update":bool)
            n321 = call "Ibeopaser.vi"("theta"=-2.5, "Hide Transparent"=w470, "Sensor [F12]"=w470) -> ("x_sensor"=w474:T6, "etc"=w472:dbl[][], "lane"=w473:dbl[][], "obs"=w475:dbl[][], "update"=w471:bool)  [unwired: 4 in]
            n322 = case shown="True" w471 {
              tunnel: w475 -> [_ w481]
              tunnel: w474 -> [_ w482]
              tunnel: w473 -> [_ w478]
              tunnel: w472 -> [_ w479]
              frame False {
              }
              frame True {
                n323 = disable-structure shown="Enabled" {
                  disable-tunnel: w481 -> [w487 w489]
                  disable-tunnel: [w486 w489] -> w480
                  disable-tunnel: w479 -> [w485 _]
                  disable-tunnel: w478 -> [w484 w488]
                  disable-tunnel: [w483 w488] -> w477
                  frame Disabled {
                    n324 = call "test3.vi"("sensor_all"=w485, "sensor_lane"=w484, "sensor_obs"=w487) -> ("lane"=w483:dbl[][], "obs"=w486:dbl[][])  [unwired: 6 in, 1 out]
                  }
                  frame Enabled {
                  }
                }
                n325 = global write "G_VEH.vi" "xsensor"(w482) -> ()
                n326 = global write "G_SEN.vi" "sensor_obs"(w480) -> ()
                n327 = global write "G_SEN.vi" "sensor_lane"(w477) -> ()
              }
            }
          }
          frame #3 {
            n328 = case shown="True" "Log" {
              frame False {
                n329 = global write "G_SEN.vi" "sensor_obs_log"(dbl[][] [] ("sensor_obs_log")) -> ()
              }
              frame True {
                n330 = global read "G_VEH.vi" "candata"() -> (w493:T8)
                n331 = Unbundle By Name(w493) -> ("VS_can"=w494:dbl)
                n332 = Not Equal To 0?(x=w494) -> (x != 0?=w492:bool)
                n333 = case shown="True" w492 {
                  frame False {
                  }
                  frame True {
                    n334 = global read "G_SEN.vi" "sensor_obs_log"() -> (w496:dbl[][])
                    n335 = global read "G_SEN.vi" "sensor_obs"() -> (w497:dbl[][])
                    n336 = call "sensor_log2.vi"("xmax"=5.0, "range^2"=16.0, "xmin"=-5.0, "FF"=0.99 ("t"), "ymin"=0.0, "ymax"=15.0, "sensor_log"=w496, "sensor_obs"=w497) -> ("sensor_log 2"=w495:dbl[][])  [unwired: 2 in, 1 out]
                    n337 = global write "G_SEN.vi" "sensor_obs_log"(w495) -> ()
                  }
                }
              }
            }
          }
        }
      }
    }
  }
